vi "myTask.vi"(8 "error in (no error)":errorcluster, 10 "stopMechanism":refnum<class "ITaskStopMechanism.lvclass">, 11 "ITask in":refnum<class "ITask.lvclass">) -> (0 "error out":errorcluster, 3 "ITask out":refnum<class "ITask.lvclass">)   [LabVIEW 2023, in "ExampleTask_MsgUserEventStop.lvclass"]
uses:
  ExampleTask_MsgUserEventStop.lvclass
  ITask/ITask.lvclass
  ITaskStopMechanism/ITaskStopMechanism.lvclass
  MsgUserEventStopMech/MsgUserEventStopMechanism.lvclass
  C:/projects/TLC_Daemon/source/ITask/ITask.lvclass
  ExampleTask_MsgUserEventStop.lvclass/ExampleTask_MsgUserEventStop.ctl
  Read description.vi
panel:
  out "receivedMessage":string="-" caption="Received message"
  out "loopCounter":i32 caption="Loop Counter"
  out "description":string
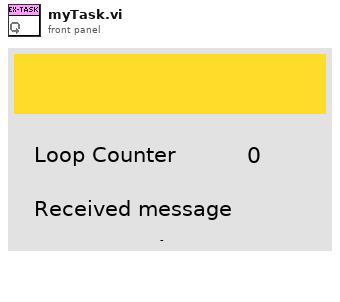
[diagram p1: front panel]
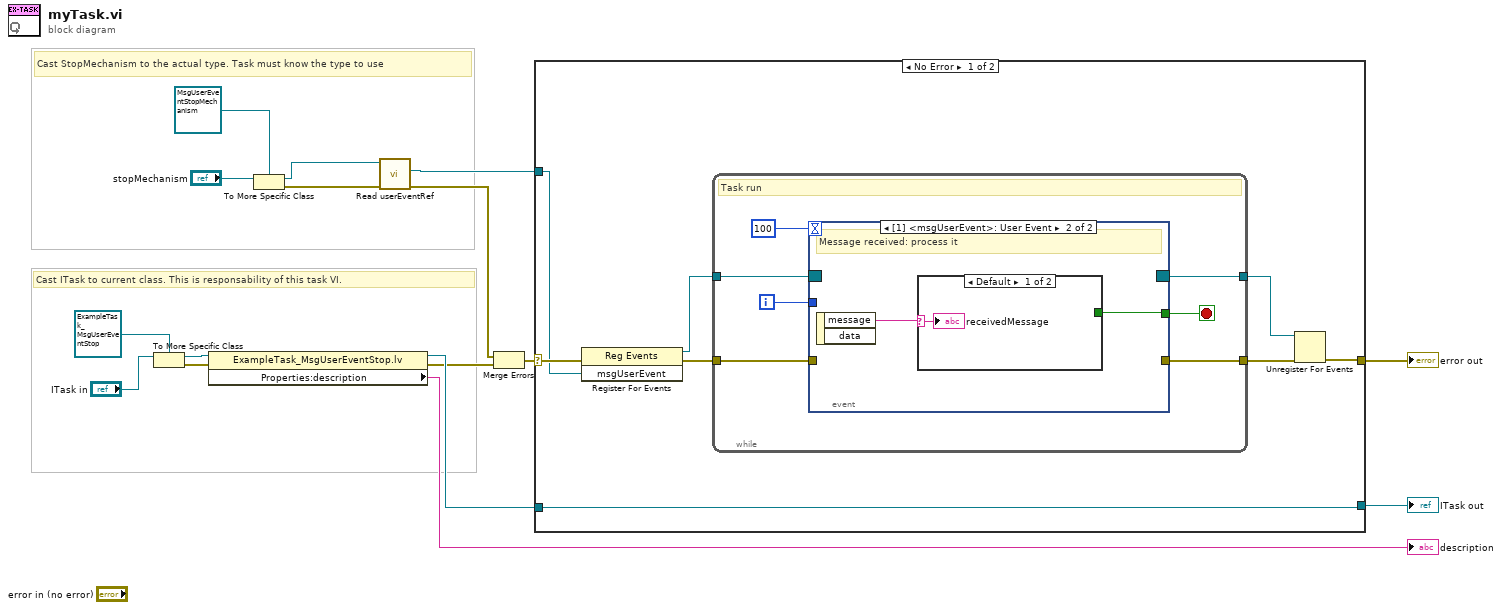
[diagram p0: block diagram]
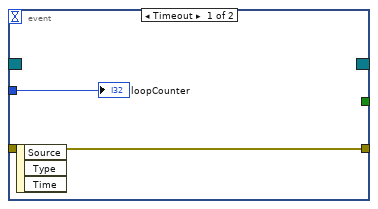
[diagram p2: hidden frame]
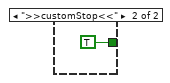
[diagram p3: hidden frame]
diagram:
  # "Cast ITask to current class. This is responsability of this task VI."
  # "Cast StopMechanism to the actual type. Task must know the type to use"
  n1 = To More Specific Class(target class=refnum<class "ExampleTask_MsgUserEventStop.lvclass"> refnum ("ExampleTask_StopNotifier.lvclass"), reference="ITask in") -> (specific class reference=w11:refnum<class "ExampleTask_MsgUserEventStop.lvclass">, error out=w12:errorcluster)  [unwired: 1 in]
  n2 = property class="ExampleTask_MsgUserEventStop.lv"(reference=w11, error in=w12) -> (reference out=w9:refnum<class "ExampleTask_MsgUserEventStop.lvclass">, error out=w7:errorcluster, "Properties:description"=→"description":string)
  n3 = To More Specific Class(target class=refnum<class "MsgUserEventStopMechanism.lvclass"> refnum ("TLC_Daemon.lvlib:NotifierStopMechanism.lvclass"), reference="stopMechanism") -> (specific class reference=w4:refnum<class "MsgUserEventStopMechanism.lvclass">, error out=w3:errorcluster)  [unwired: 1 in]
  n4 = call "Read userEventRef.vi"("error in (no error)"=w3, "MsgUserEventStopMechanism In"=w4) -> ("error out"=w2:errorcluster, "msgUserEvent"=w1:refnum<user-event>)  [unwired: 7 in, 1 out]
  n5 = Merge Errors(w2, w7) -> (w6:errorcluster)
  n6 = case shown="No Error" w6 {
    selector: w6 -> [w23 w39]
    tunnel: w1 -> [w17 _]
    tunnel: w9 -> [w24 w38]
    tunnel: [w24 w38] -> w8
    tunnel: [w19 w39] -> w5
    frame No Error {
      n7 = register-events(error in=w23, w17) -> (reference out=w21:refnum<event-registration>, error out=w22:errorcluster)  [unwired: 1 in]
      n8 = while {
        tunnel: w22 -> [w31]
        tunnel: [w30] -> w18
        tunnel: w21 -> [w27]
        tunnel: [w25] -> w20
        i -> [w29]
        stop <- w26 stop-if-true
        # "Task run"
        n9 = event shown="[1] <msgUserEvent>: User Event" {
          selector: w27 -> [_ _]
          dyn-events: [_ _] -> w25
          timeout: 100 -> [_ _]
          tunnel: w31 -> [w33 _]
          tunnel: [w33 _] -> w30
          tunnel: w29 -> [w32 _]
          tunnel: [_ w34] -> w26
          event Timeout {
            n10 = event-data() -> ()  [unwired: 1 in, 3 out]
            "loopCounter" <- w32
          }
          event User Event {
            # "Message received: process it"
            n11 = event-data() -> ("message"=w35:string)  [unwired: 1 in, 1 out]
            n12 = case shown="Default" w35 {
              selector: w35 -> [w36 _]
              tunnel: [_ TRUE] -> w34
              frame Default {
                "receivedMessage" <- w36
              }
              frame ">>customStop<<" {
              }
            }
          }
        }
      }
      n13 = Unregister For Events(event registration refnum=w20, error in=w18) -> (error out=w19:errorcluster)
    }
    frame Error {
    }
  }
  "error out" <- w5
  "ITask out" <- w8
